vi "to_dom.vi"() -> ()   [LabVIEW 2017]
uses:
  <vilib>/userdefined/High Color/IMAQdx.ctl
  <vilib>/myRIO/Instrument Drivers/Onboard IO/DIO/typedefs/DIO Reference.ctl
  <vilib>/myRIO/Common/Instrument Driver Framework/Utilities/typedefs/myRIO Generic Hardware Reference.ctl
  <vilib>/myRIO/Common/Instrument Driver Framework/Utilities/typedefs/Hardware Version Enum.ctl
  <vilib>/myRIO/Common/Instrument Driver Framework/Utilities/typedefs/myRIO v1.0 Reference.ctl
  <vilib>/myRIO/Common/Instrument Driver Framework/Utilities/typedefs/Generic FPGA Reference.ctl
  <vilib>/myRIO/Common/Instrument Driver Framework/myRIO v1.0/DIO/typedefs/DIO Channels List.ctl
  <vilib>/myRIO/Common/Instrument Driver Framework/myRIO v1.0/DIO/typedefs/DIO Channels Enum.ctl
  <vilib>/userdefined/High Color/nirio_resource_hc.ctl
  <vilib>/myRIO/Common/Instrument Driver Framework/Utilities/vis/Is FPGA Ref Available.vi
  <vilib>/myRIO/Common/Instrument Driver Framework/myRIO v1.0/DIO/vis/myRIO v1.1 Open DIO.vi
  <vilib>/myRIO/Instrument Drivers/Onboard IO/DIO/vis/Write.vi
  <vilib>/myRIO/Common/Instrument Driver Framework/Utilities/vis/Validate Channels.vi
  <vilib>/myRIO/Common/Instrument Driver Framework/myRIO v1.0/DIO/vis/myRIO v1.0 Reserve DIO.vi
  <vilib>/myRIO/Common/Instrument Driver Framework/myRIO v1.0/Resource Manager/vis/myRIO v1.0 Reserve Channel List.vi
  <vilib>/myRIO/Common/Instrument Driver Framework/myRIO v1.0/DIO/vis/myRIO v1.0 Build MUX Configuration DIO.vi
  <vilib>/myRIO/Common/Instrument Driver Framework/myRIO v1.0/Resource Manager/vis/myRIO v1.0 Reserve Channel.vi
  <vilib>/myRIO/Common/Instrument Driver Framework/myRIO v1.0/Resource Manager/vis/myRIO v1.0 Unreserve Channel.vi
  <vilib>/myRIO/Common/Instrument Driver Framework/myRIO v1.0/Resource Manager/vis/myRIO v1.0 Create Configuration List.vi
  <vilib>/myRIO/Common/Instrument Driver Framework/myRIO v1.0/Resource Manager/vis/myRIO v1.0 Build Mutex Name.vi
  <vilib>/Utility/VariantDataType/GetNumericInfo.vi
  <vilib>/Utility/error.llb/Error Cluster From Error Code.vi
  <vilib>/myRIO/Common/Instrument Driver Framework/myRIO v1.0/myRIO v1.1 Open.vi
  <vilib>/myRIO/Common/Instrument Driver Framework/Utilities/vis/IO Manager.vi
  <vilib>/myRIO/Common/Instrument Driver Framework/Utilities/vis/Configuration Manager.vi
  <vilib>/myRIO/Common/Instrument Driver Framework/myRIO v1.0/Resource Manager/vis/myRIO v1.0 Configure IO.vi
  <vilib>/myRIO/Common/Instrument Driver Framework/myRIO v1.0/myRIO v1.0 Close.vi
  <vilib>/myRIO/Common/Instrument Driver Framework/myRIO v1.0/DIO/vis/myRIO v1.0 Write DIO.vi
  <vilib>/myRIO/Express VI/Onboard Devices/LED/LED Express VI.xnode
  <vilib>/myRIO/Instrument Drivers/Onboard IO/DIO/vis/myRIO DIO Open.xnode
  <vilib>/vision/driver/NI_Vision_Acquisition_Software.lvlib
  <vilib>/myRIO/Instrument Drivers/Onboard IO/DIO/DIO.lvlib
panel:
  out "X 2":sgl
  out "zelenka 2":string
  out "X":sgl
  out "zelenka":string
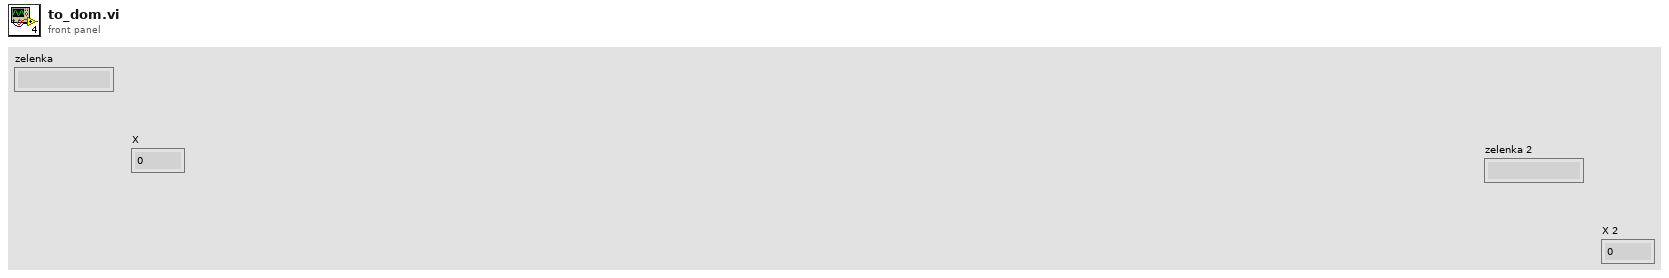
[diagram p1: front panel]
types:
  T1 = typedef "IMAQdx.ctl" = refnum<k21>
  T2 = typedef "DIO.lvlib/DIO Reference.ctl" = cluster{"myRIO Reference":T3, "DIO Channels List":T7}
  T3 = typedef "myRIO Generic Hardware Reference.ctl" = cluster{"myRIO Model":T4, "myRIO Hardware Reference":T5}
  T4 = typedef "Hardware Version Enum.ctl" = enum16{"Unknown", "myRIO-1900", "myRIO-1950", "roboRIO", "NI ELVIS RIO CM"}
  T5 = typedef "myRIO v1.0 Reference.ctl" = cluster{"Generic FPGA Reference":T6, "Allow multiple opens":bool}
  T6 = typedef "Generic FPGA Reference.ctl" = refnum<k20>
  T7 = typedef "DIO Channels List.ctl" = T8[]
  T8 = typedef "DIO Channels Enum.ctl" = enum16{"Not Connected", "C/DIO0", "C/DIO1", "C/DIO2", "C/DIO3", "C/DIO4", "C/DIO5", "C/DIO6", "C/DIO7", "A/DIO0", "A/DIO1", "A/DIO2", "A/DIO3", "A/DIO4", "A/DIO5", "A/DIO6", "A/DIO7", "A/DIO8", "A/DIO9", "A/DIO10", "A/DIO11", "A/DIO12", "A/DIO13", "A/DIO14", "A/DIO15", "B/DIO0", "B/DIO1", "B/DIO2", "B/DIO3", "B/DIO4", "B/DIO5", "B/DIO6", "B/DIO7", "B/DIO8", "B/DIO9", "B/DIO10", "B/DIO11", "B/DIO12", "B/DIO13", "B/DIO14", "B/DIO15", "LED0", "LED1", "LED2", "LED3", "Button0", "DIO/DIO0", "DIO/DIO1", "DIO/DIO2", "DIO/DIO3", "DIO/DIO4", "DIO/DIO5", "DIO/DIO6", "DIO/DIO7", "DIO/DIO8", "DIO/DIO9", "SPI/CS0", "SPI/CS1", "SPI/CS2", "SPI/CS3", "LED RADIO (Green)", "LED RADIO (Red)", "LED COMM (Green)", "LED COMM (Red)", "LED MODE (Green)", "LED MODE (Red)"}
  T9 = typedef "nirio_resource_hc.ctl" = tag
  T10 = typedef "IMAQ Image.ctl" = refnum<image>
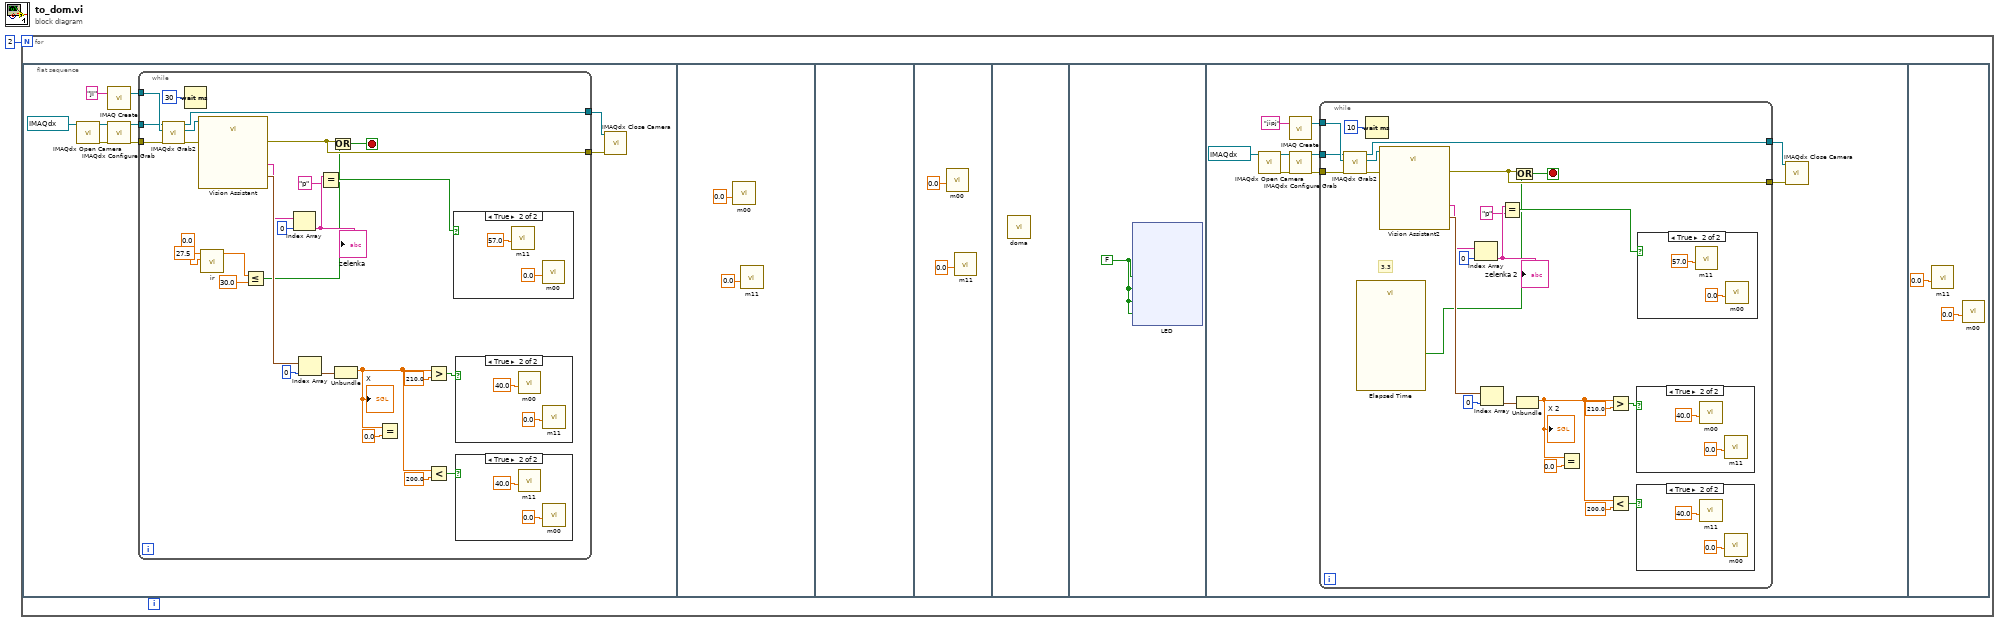
[diagram p0: block diagram]
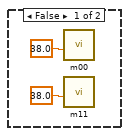
[diagram p3: hidden frame]
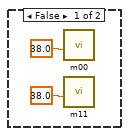
[diagram p4: hidden frame]
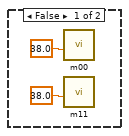
[diagram p6: hidden frame]
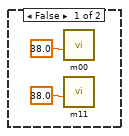
[diagram p7: hidden frame]
diagram:
  n1 = for {
    N: 2 -> [_]
    n2 = flat-sequence {
      frame #0 {
        n3 = call <vilib>:"IMAQdx Open Camera.vi"("Session In"=T1 "cam1") -> ("error out"=w7:errorcluster, "Session Out"=w6:T1)  [unwired: 9 in]
        n4 = call "IMAQ Create"("Image Name"="ji") -> ("New Image"=w4:T10)  [unwired: 4 in, 1 out]
        n5 = call <vilib>:"IMAQdx Configure Grab.vi"("error in"=w7, "Session In"=w6) -> ("error out"=w8:errorcluster, "Session Out"=w5:T1)  [unwired: 8 in]
        n6 = while {
          tunnel: w8 -> [w33]
          tunnel: w4 -> [w32]
          tunnel: w5 -> [w31]
          tunnel: [w30] -> w10
          tunnel: [w29] -> w9
          stop <- w11 stop-if-true
          n7 = call <vilib>:"IMAQdx Grab2.vi"("error in"=w33, "Image In"=w32, "Session In"=w31) -> ("error out"=w35:errorcluster, "Image Out"=w34:T10, "Session Out"=w30:T1)  [unwired: 5 in, 1 out]
          n8 = Wait (ms)(milliseconds to wait=u32 30) -> ()  [unwired: 1 out]
          n9 = call "Vision Assistant"("Image In"=w34, "error in"=w35) -> ("Edges Coordinates (Edge Detector 1)"=w38:cluster{"X":sgl, "Y":sgl}[], "Classes (Color Classification 1)"=w21:string[], "error out"=w29:errorcluster)  [unwired: 22 in, 1 out]
          n10 = call "ir.vi"("Koffset [cm]"=0.0, "Kscale [cm-V]"=27.5) -> ("см"=w16:dbl)  [unwired: 8 in, 1 out]
          n11 = Less Or Equal?(x=w16, y=30.0) -> (x <= y?=w12:bool)
          n12 = Index Array(array=w21, index=0) -> (element=w19:string)
          "zelenka" <- w19
          n13 = Index Array(array=w38, index=0) -> (element=w37:cluster{"X":sgl, "Y":sgl})
          n14 = Equal?(x=w19, y="p") -> (x = y?=w17:bool)
          n15 = Or(x=w29, y=w12) -> (x .or. y?=w11:bool)
          n16 = Unbundle(w37) -> ("X"=w24:sgl)  [unwired: 1 out]
          "X" <- w24
          n17 = Equal?(x=w24, y=sgl 0.0) -> ()  [unwired: 1 out]
          n18 = Greater?(x=w24, y=sgl 210.0) -> (0:w27:bool)
          n19 = Less?(x=w24, y=sgl 200.0) -> (x < y?=w23:bool)
          n20 = case shown="True" w17 {
            frame False {
            }
            frame True {
              n21 = call "m11.vi"("position"=57.0) -> ()  [unwired: 10 in, 1 out]
              n22 = call "m00.vi"("position"=0.0) -> ()  [unwired: 10 in, 1 out]
            }
          }
          n23 = case shown="True" w27 {
            frame False {
              n24 = call "m00.vi"("position"=38.0) -> ()  [unwired: 10 in, 1 out]
              n25 = call "m11.vi"("position"=38.0) -> ()  [unwired: 10 in, 1 out]
            }
            frame True {
              n26 = call "m00.vi"("position"=40.0) -> ()  [unwired: 10 in, 1 out]
              n27 = call "m11.vi"("position"=0.0) -> ()  [unwired: 10 in, 1 out]
            }
          }
          n28 = case shown="True" w23 {
            frame False {
              n29 = call "m00.vi"("position"=38.0) -> ()  [unwired: 10 in, 1 out]
              n30 = call "m11.vi"("position"=38.0) -> ()  [unwired: 10 in, 1 out]
            }
            frame True {
              n31 = call "m11.vi"("position"=40.0) -> ()  [unwired: 10 in, 1 out]
              n32 = call "m00.vi"("position"=0.0) -> ()  [unwired: 10 in, 1 out]
            }
          }
        }
        n33 = call <vilib>:"IMAQdx Close Camera.vi"("error in"=w9, "Session In"=w10) -> ()  [unwired: 9 in, 1 out]
      }
      frame #1 {
        n34 = call "m00.vi"("position"=0.0) -> ()  [unwired: 10 in, 1 out]
        n35 = call "m11.vi"("position"=0.0) -> ()  [unwired: 10 in, 1 out]
      }
      frame #2 {
      }
      frame #3 {
        n36 = call "m00.vi"("position"=0.0) -> ()  [unwired: 10 in, 1 out]
        n37 = call "m11.vi"("position"=0.0) -> ()  [unwired: 10 in, 1 out]
      }
      frame #4 {
        n38 = call "doma.vi"() -> ()  [unwired: 12 in]
      }
      frame #5 {
        w53 = FALSE
        n39 = xnode "LED"("LED0"=w53, "LED1"=w53, "LED2"=w53, "LED3"=w53) -> ()  [unwired: 1 in, 1 out]
      }
      frame #6 {
        n40 = call <vilib>:"IMAQdx Open Camera.vi"("Session In"=T1 "cam1") -> ("error out"=w97:errorcluster, "Session Out"=w96:T1)  [unwired: 9 in]
        n41 = call "IMAQ Create"("Image Name"="jipj") -> ("New Image"=w94:T10)  [unwired: 4 in, 1 out]
        n42 = call <vilib>:"IMAQdx Configure Grab.vi"("error in"=w97, "Session In"=w96) -> ("error out"=w98:errorcluster, "Session Out"=w95:T1)  [unwired: 8 in]
        n43 = while {
          tunnel: w98 -> [w119]
          tunnel: w94 -> [w118]
          tunnel: w95 -> [w117]
          tunnel: [w116] -> w100
          tunnel: [w115] -> w99
          stop <- w102 stop-if-true
          # "3,3"
          n44 = call <vilib>:"IMAQdx Grab2.vi"("error in"=w119, "Image In"=w118, "Session In"=w117) -> ("error out"=w121:errorcluster, "Image Out"=w120:T10, "Session Out"=w116:T1)  [unwired: 5 in, 1 out]
          n45 = call "Elapsed Time"() -> ("Time has Elapsed"=w101:bool)  [unwired: 12 in, 7 out]
          n46 = Wait (ms)(milliseconds to wait=u32 10) -> ()  [unwired: 1 out]
          n47 = call "Vision Assistant2"("Image In"=w120, "error in"=w121) -> ("Edges Coordinates (Edge Detector 1)"=w124:cluster{"X":sgl, "Y":sgl}[], "Classes (Color Classification 1)"=w107:string[], "error out"=w115:errorcluster)  [unwired: 22 in, 1 out]
          n48 = Index Array(array=w107, index=0) -> (element=w105:string)
          "zelenka 2" <- w105
          n49 = Index Array(array=w124, index=0) -> (element=w123:cluster{"X":sgl, "Y":sgl})
          n50 = Equal?(x=w105, y="p") -> (x = y?=w103:bool)
          n51 = Or(x=w115, y=w101) -> (x .or. y?=w102:bool)
          n52 = Unbundle(w123) -> ("X"=w110:sgl)  [unwired: 1 out]
          "X 2" <- w110
          n53 = Equal?(x=w110, y=sgl 0.0) -> ()  [unwired: 1 out]
          n54 = Greater?(x=w110, y=sgl 210.0) -> (0:w113:bool)
          n55 = Less?(x=w110, y=sgl 200.0) -> (x < y?=w109:bool)
          n56 = case shown="True" w113 {
            frame False {
              n57 = call "m00.vi"("position"=38.0) -> ()  [unwired: 10 in, 1 out]
              n58 = call "m11.vi"("position"=38.0) -> ()  [unwired: 10 in, 1 out]
            }
            frame True {
              n59 = call "m00.vi"("position"=40.0) -> ()  [unwired: 10 in, 1 out]
              n60 = call "m11.vi"("position"=0.0) -> ()  [unwired: 10 in, 1 out]
            }
          }
          n61 = case shown="True" w109 {
            frame False {
              n62 = call "m00.vi"("position"=38.0) -> ()  [unwired: 10 in, 1 out]
              n63 = call "m11.vi"("position"=38.0) -> ()  [unwired: 10 in, 1 out]
            }
            frame True {
              n64 = call "m11.vi"("position"=40.0) -> ()  [unwired: 10 in, 1 out]
              n65 = call "m00.vi"("position"=0.0) -> ()  [unwired: 10 in, 1 out]
            }
          }
          n66 = case shown="True" w103 {
            frame False {
            }
            frame True {
              n67 = call "m11.vi"("position"=57.0) -> ()  [unwired: 10 in, 1 out]
              n68 = call "m00.vi"("position"=0.0) -> ()  [unwired: 10 in, 1 out]
            }
          }
        }
        n69 = call <vilib>:"IMAQdx Close Camera.vi"("error in"=w99, "Session In"=w100) -> ()  [unwired: 9 in, 1 out]
      }
      frame #7 {
        n70 = call "m11.vi"("position"=0.0) -> ()  [unwired: 10 in, 1 out]
        n71 = call "m00.vi"("position"=0.0) -> ()  [unwired: 10 in, 1 out]
      }
    }
  }
